vi "UI.vi"(8 "error in (no error)":errorcluster, 11 "Callback Producer in":refnum<class "Callback Producer.lvclass">) -> (0 "error out":errorcluster, 3 "Callback Producer out":refnum<class "Callback Producer.lvclass">)   [LabVIEW 2012, in "Callback Producer.lvclass"]
uses:
  Callback Producer.lvclass
panel:
  in  "Do Callback":bool
  in  "Numeric":dbl
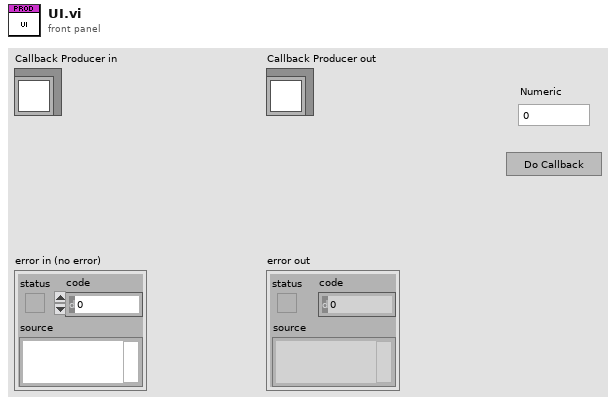
[diagram p1: front panel]
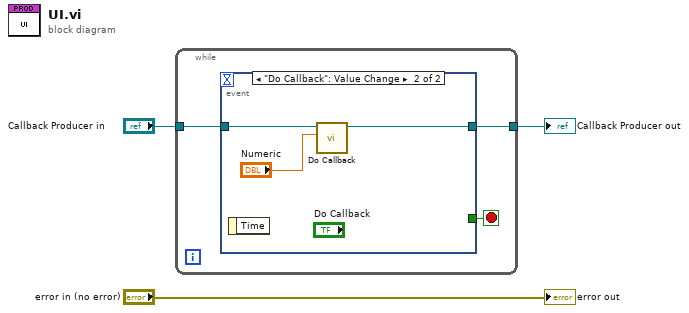
[diagram p0: block diagram]
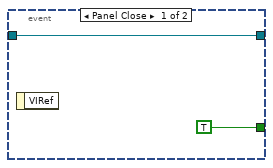
[diagram p2: hidden frame]
diagram:
  n1 = while {
    tunnel: "Callback Producer in" -> [w6]
    tunnel: [w4] -> w1
    stop <- w5 stop-if-true
    n2 = event shown="[1] \"Do Callback\": Value Change" {
      selector: _ -> [_ _]
      dyn-events: _ -> [_ _]
      timeout: _ -> [_ _]
      tunnel: w6 -> [w7 w11]
      tunnel: [TRUE _] -> w5
      tunnel: [w7 w9] -> w4
      event Panel Close {
        n3 = event-data() -> ()  [unwired: 1 in, 1 out]
      }
      event "Do Callback": Value Change {
        n4 = event-data() -> ()  [unwired: 1 in, 1 out]
        n5 = call "Do Callback.vi"("Numeric"="Numeric", "Callback Producer in"=w11) -> ("Callback Producer out"=w9:refnum<class "Callback Producer.lvclass">)  [unwired: 8 in, 1 out]
      }
    }
  }
  "Callback Producer out" <- w1
  "error out" <- "error in (no error)"
